vi "get_SampleHandler_state.vi"(8 "error in (no error)":errorcluster caption="エラー入力（エラーなし）", 11 "VISAリソース名":refnum<visa-resource-name>) -> (0 "error out":errorcluster caption="エラー出力", 2 "response":string, 3 "VISAリソース名（出力）":refnum<visa-resource-name>)   [LabVIEW 2017]
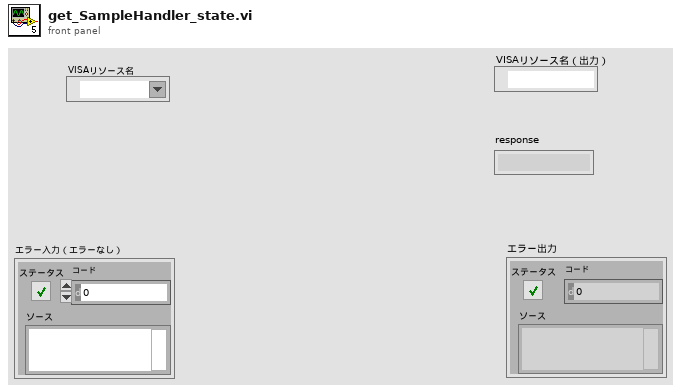
[diagram p1: front panel]
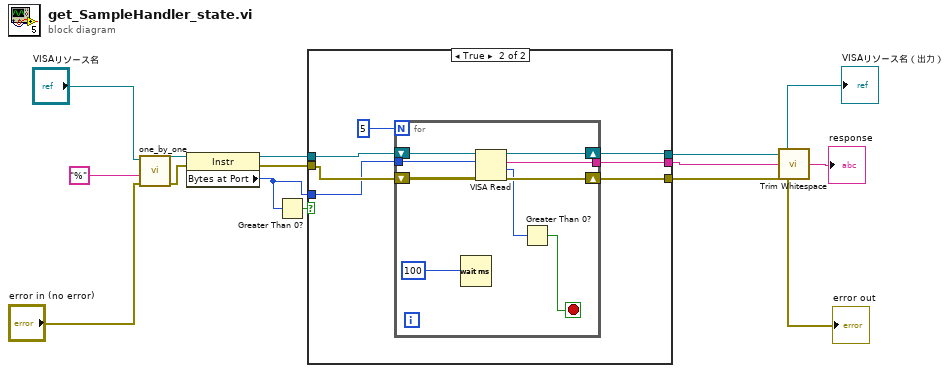
[diagram p0: block diagram]
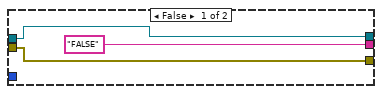
[diagram p2: hidden frame]
diagram:
  n1 = call "one_by_one.vi"("error in (no error)"="error in (no error)", "入力文字"="%", "VISAリソース名"="VISAリソース名") -> ("error out"=w11:errorcluster, "VISAリソース名出力"=w12:refnum<visa-resource-name>)  [unwired: 7 in]
  n2 = property class="Instr"(reference=w12, error in=w11) -> (reference out=w10:refnum<visa-resource-name>, error out=w9:errorcluster, "Bytes at Port"=w3:u32)
  n3 = Greater Than 0?(x=w3) -> (x > 0?=w8:bool)
  n4 = case shown="TRUE" w8 {
    tunnel: [w15 w23] -> w4
    tunnel: ["FALSE" w22] -> w1
    tunnel: [w14 w21] -> w5
    tunnel: w10 -> [w15 w20]
    tunnel: w9 -> [w14 w19]
    tunnel: w3 -> [_ w17]
    frame False {
    }
    frame True {
      n5 = for {
        N: 5 -> [_]
        tunnel: [w31] -> w22
        tunnel: w17 -> [w27]
        shift-right: [w32] -> w23
        shift-left: w20 -> [w29]
        shift-right: [w30] -> w21
        shift-left: w19 -> [w28]
        stop <- w24 stop-if-true
        n6 = Wait (ms)(milliseconds to wait=100) -> ()  [unwired: 1 out]
        n7 = VISA Read(VISA resource name=w29, byte count=w27, error in (no error)=w28) -> (VISA resource name out=w32:refnum<visa-resource-name>, read buffer=w31:string, return count=w25:u32, error out=w30:errorcluster)
        n8 = Greater Than 0?(x=w25) -> (x > 0?=w24:bool)
      }
    }
  }
  "VISAリソース名（出力）" <- w4
  "error out" <- w5
  n9 = call <vilib>:"Trim Whitespace.vi"("string"=w1) -> ("trimmed string"=→"response":string)  [unwired: 1 in]
